vi "Median.vi"(0 "X":dbl[](array[numeric]) format="%0.2f") -> (1 "median":dbl format="%0.2f", 2 "error":i32)   [LabVIEW 2017, in "NI_AALBase.lvlib"]
doc: "Finds the median value of the input sequence <B>X</B> by sorting the values of <B>X</B> and averaging the middle element(s) of the sorted array."
uses:
  <vilib>/Analysis/NI_AALBase.lvlib
  <resource>/lvanlys.dll
panel:
  # "Median"
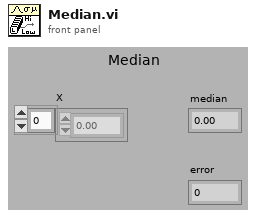
[diagram p1: front panel]
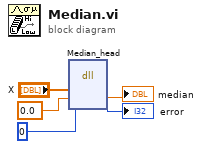
[diagram p0: block diagram]
diagram:
  n1 = dll-call lib="e:/builds/penguin/labview/branches/2017/dev/dist/resource/lvanlys.*" fn="Median_head"("X"="X", "output param"=0.0, "output param"=0) -> ("output param"=→"median":dbl, "output param"=→"error":i32)  [unwired: 5 in, 2 out]
